vi "tcvInit.vi"(8 "error in":errorcluster, 11 "devices":T1) -> (0 "error out":errorcluster, 2 "SetDevice":string, 3 "tcv out":refnum<class "tcv.lvclass">)   [LabVIEW 2025, in "tcv.lvlib" / "tcv.lvclass"]
uses:
  tcv.lvclass
  tcv.lvclass/tcv.ctl
  def/devices.ctl
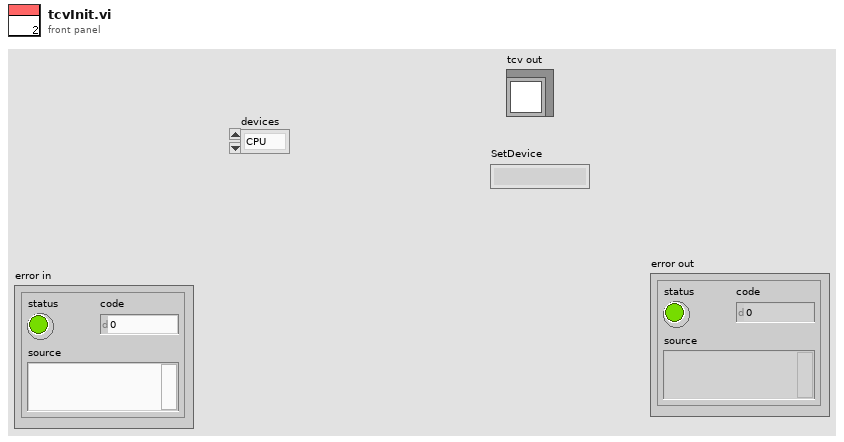
[diagram p1: front panel]
types:
  T1 = typedef "tcv.lvlib/tcv.lvclass/devices.ctl" = enum16{"CPU", "GPU0"}
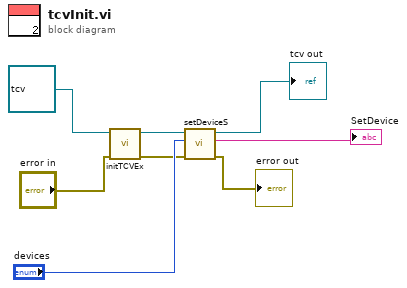
[diagram p0: block diagram]
diagram:
  n1 = call-dynamic "initTCVEx.vi"("error in (no error)"="error in", "tcv in"=refnum<class "tcv.lvclass"> refnum) -> ("error out"=w4:errorcluster, "tcv out"=w5:refnum<class "tcv.lvclass">)  [unwired: 8 in]
  n2 = call-dynamic "setDeviceS.vi"("error in (no error)"=w4, "devices"="devices", "tcv in"=w5) -> ("error out"=→"error out":errorcluster, "SetDevice"=→"SetDevice":string, "tcv out"=→"tcv out":refnum<class "tcv.lvclass">)  [unwired: 6 in]
